vi "SDO data conversion.vi"(11 "Decimal Input":i32) -> (2 "Array":u8[](array[numeric]), 3 "String":string)   [LabVIEW 2018]
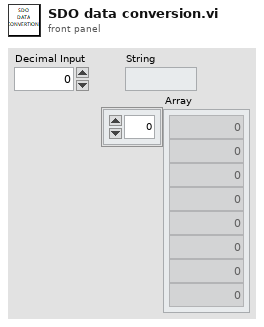
[diagram p1: front panel]
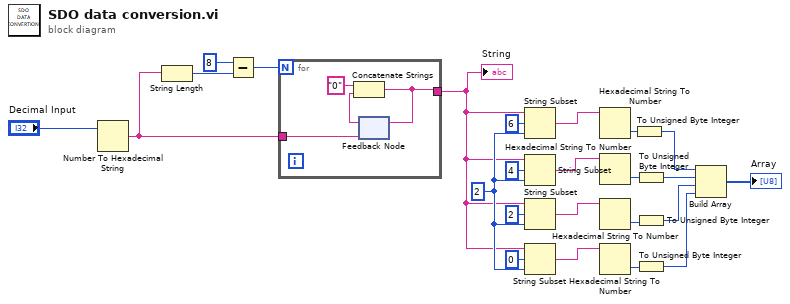
[diagram p0: block diagram]
diagram:
  w10 = 2 ("length (rest)")
  n1 = Number To Hexadecimal String(2:"Decimal Input") -> (0:w1:string)  [unwired: 1 in]
  n2 = String Length(string=w1) -> (length=w2:i32)
  n3 = Subtract(x=8, y=w2) -> (x-y=w3:i32)
  n4 = for {
    N: w3 -> [_]
    tunnel: w1 -> [w26]
    tunnel: [w25] -> w9
    n5 = feedback #1(w26) -> (w27:string)
    n6 = Concatenate Strings("0" ("string"), w27) -> (w25:string)
    n7 = feedback-in #1(w25) -> ()
  }
  "String" <- w9
  n8 = String Subset(string=w9, offset (0)=6, length (rest)=w10) -> (substring=w11:string)
  n9 = String Subset(string=w9, offset (0)=4, length (rest)=w10) -> (substring=w12:string)
  n10 = String Subset(string=w9, offset (0)=2, length (rest)=w10) -> (substring=w13:string)
  n11 = String Subset(string=w9, offset (0)=0, length (rest)=w10) -> (substring=w14:string)
  n12 = Hexadecimal String To Number(string=w11) -> (number=w15:u32)  [unwired: 2 in, 1 out]
  n13 = Hexadecimal String To Number(string=w12) -> (number=w16:u32)  [unwired: 2 in, 1 out]
  n14 = Hexadecimal String To Number(string=w13) -> (number=w17:u32)  [unwired: 2 in, 1 out]
  n15 = Hexadecimal String To Number(string=w14) -> (number=w18:u32)  [unwired: 2 in, 1 out]
  n16 = To Unsigned Byte Integer(number=w15) -> (unsigned 8bit integer=w20:u8)
  n17 = To Unsigned Byte Integer(number=w16) -> (unsigned 8bit integer=w21:u8)
  n18 = To Unsigned Byte Integer(number=w17) -> (unsigned 8bit integer=w22:u8)
  n19 = To Unsigned Byte Integer(number=w18) -> (unsigned 8bit integer=w23:u8)
  n20 = Build Array(w20, w21, w22, w23) -> (→"Array":u8[])
